vi "Convert plane.vi"(7 "File Handle":u32, 8 "error in (no error)":errorcluster, 9 "Frame Index":i32=-1, 10 "file in":path, 11 "Image in":T1) -> (0 "error out":errorcluster, 3 "Image out":T1)   [LabVIEW 2012, in "DAQOrcaFlash.lvclass"]
uses:
  DAQOrcaFlash.lvclass
  <vilib>/vision/Image Controls.llb/IMAQ Image.ctl
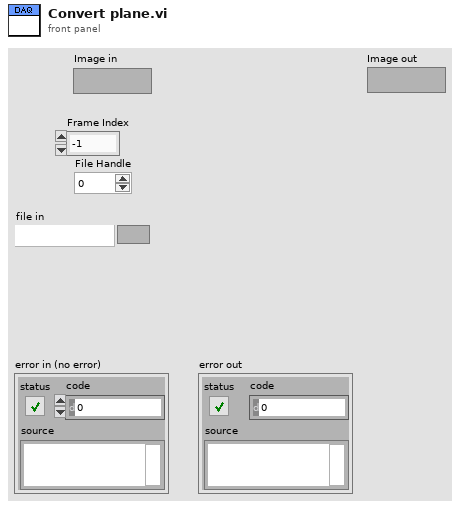
[diagram p1: front panel]
types:
  T1 = typedef "IMAQ Image.ctl" = refnum<image>
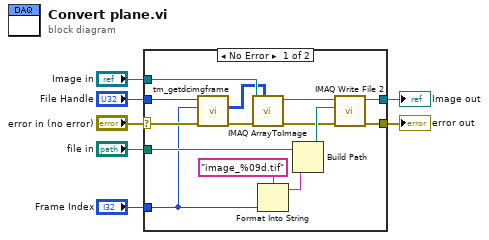
[diagram p0: block diagram]
diagram:
  n1 = case shown="No Error" "error in (no error)" {
    selector: "error in (no error)" -> [w19 w23]
    tunnel: "File Handle" -> [w21 _]
    tunnel: "file in" -> [w13 _]
    tunnel: [w17 w23] -> w5
    tunnel: "Frame Index" -> [w12 _]
    tunnel: "Image in" -> [w18 w22]
    tunnel: [w16 w22] -> w2
    frame No Error {
      n2 = call <userlib>:"tm_getdcimgframe.vi"("error in (no error)"=w19, "Frame Index"=w12, "File Handle in"=w21) -> ("error out"=w9:errorcluster, "Data"=w10:u16[][])  [unwired: 5 in, 2 out]
      n3 = call "IMAQ ArrayToImage"("Image Pixels (U16)"=w10, "error in (no error)"=w9, "Image"=w18) -> ("error out"=w8:errorcluster, "Image Out"=w11:T1)  [unwired: 7 in]
      n4 = Format Into String(format string="image_%09d.tif", w12) -> (resulting string=w14:string)  [unwired: 2 in, 1 out]
      n5 = Build Path(base path=w13, name or relative path=w14) -> (appended path=w20:path)
      n6 = call-poly "IMAQ Write File 2"("error in (no error)"=w8, "File Path"=w20, "Image"=w11) -> ("error out"=w17:errorcluster, "Image Out (duplicate)"=w16:T1)  [unwired: 7 in]
    }
    frame Error {
    }
  }
  "error out" <- w5
  "Image out" <- w2
